vi "ex7-17.vi"() -> ()   [LabVIEW 2013]
panel:
  out "String":string
  out "Boolean":bool
  out "Numeric 2":dbl
  out "Numeric":dbl
  in  "Cluster":T1
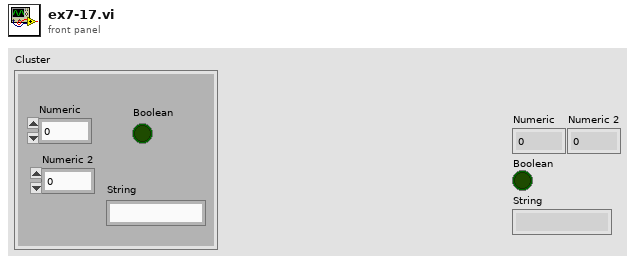
[diagram p1: front panel]
types:
  T1 = cluster{"Numeric":dbl, "Numeric 2":dbl, "Boolean":bool, "String":string}
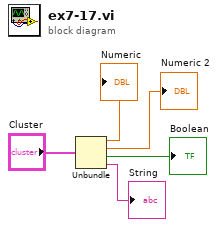
[diagram p0: block diagram]
diagram:
  n1 = Unbundle("Cluster") -> ("Numeric"=→"Numeric":dbl, "Numeric 2"=→"Numeric 2":dbl, "Boolean"=→"Boolean":bool, "String"=→"String":string)
